vi "SetNumberKineticsSD.vi"(2 "error in (no error)":errorcluster, 3 "number":i32) -> (0 "error out":errorcluster, 1 "DLL error code":u32)   [LabVIEW 2015]
doc: "This function will set the number of scans (possibly accumulated scans) to be taken during a single acquisition sequence. This will only take effect if the acquisition mode is Kinetic Series.\n\n<B>Parameter:</B>\nnumber - number of scans to store\n\n<B>Error codes:</B>\nDRV_SUCCESS - Series length set.\nDRV_NOT_INITIALIZED - System not initialized.\nDRV_ACQUIRING - Acquisition in progress.\nDRV_P1INVALID - Number in series invalid."
uses:
  DLL/atmcd32d.dll
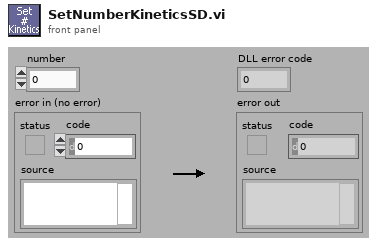
[diagram p1: front panel]
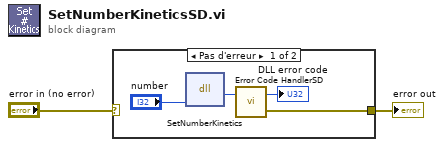
[diagram p0: block diagram]
diagram:
  n1 = case shown="Pas d'erreur" "error in (no error)" {
    selector: "error in (no error)" -> [_ w7]
    tunnel: [w5 w7] -> w1
    frame No Error {
      n2 = dll-call lib="G:/SD/TRANCON-2015/DLL/Atmcd32d.dll" fn="SetNumberKinetics"("number"="number") -> (w6:u32)  [unwired: 4 in, 2 out]
      n3 = call "Error Code HandlerSD.vi"("DLL error code"=w6) -> ("error out"=w5:errorcluster, "dup DLL error code"=→"DLL error code":u32)  [unwired: 1 in]
    }
    frame Error {
    }
  }
  "error out" <- w1
